vi "Autonomous Independent.vi"() -> ()   [LabVIEW 2013]
doc: "This VI is called when autonomous begins, and will automatically be terminated when autonomous ends. You can carry out timed or sensor driven robot movement independently without needing to return to the caller."
uses:
  Robot Global Data.vi
  <vilib>/Rock Robotics/WPI/RobotDrive/WPI_RobotDriveArcadeDrive_Standard(NoSaturation).vi
  <vilib>/Rock Robotics/WPI/RobotDrive/WPI_RobotDriveGetSetRefNum.vi
  <vilib>/Rock Robotics/WPI/Joystick/WPI_JoystickGetSetRefNum.vi
panel:
  out "Current Movement, for debugging":T1 {"Y Joystick Value" scale=1.0..-1.0; "X Joystick Value" scale=-1.0..1.0}
  in  "Array of robot movements":T2(array[cluster]) {"Y Joystick Value" scale=1.0..-1.0; "X Joystick Value" scale=-1.0..1.0}
  # "Be sure to right-click and choose Data Operations>>Make Current Value default if you want to save the array values with the VI"
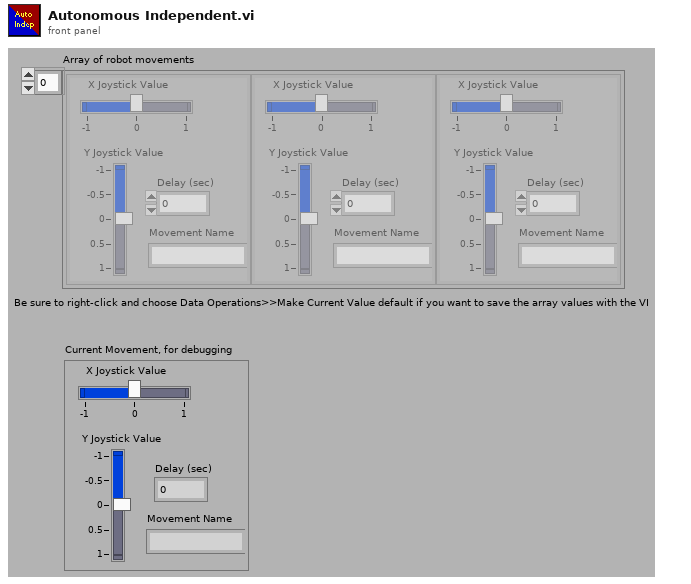
[diagram p1: front panel]
types:
  T1 = cluster{"X Joystick Value":dbl, "Y Joystick Value":dbl, "Delay (sec)":dbl, "Movement Name":string}
  T2 = cluster{"X Joystick Value":dbl, "Y Joystick Value":dbl, "Delay (sec)":dbl, "Movement Name":string}[]
  T3 = typedef "WPI_JoystickDevRef.ctl" = cluster{"Device":T4}
  T4 = typedef "WPI_JoystickDeviceEnum.ctl" = enum16{"USB 1", "USB 2", "USB 3", "USB 4", "Kinect 1", "Kinect 2"}
  T5 = cluster{"axis 1 (x)":dbl, "axis 2 (y)":dbl, "axis 3 (throttle)":dbl, "axis 4":dbl, "axis 5":dbl, "axis 6":dbl}
  T6 = typedef "WPI_RobotDriveDevRef.ctl" = cluster{"DevStatus":errorcluster, "Motors[]":T7[], "Square Inputs":bool, "Max Output":dbl, "Isochronous":bool}
  T7 = typedef "WPI_MotorControlDeviceRef.ctl" = cluster{"DeviceStatus":errorcluster, "Type":enum16{"PWM", "CAN"}, "PWM":cluster{"Digital Module":T8, "PWM Channel":T9, "DeadBand":T10}, "CAN":cluster{"Device Number":u8, "Control Mode":T11, "Semaphore":T12, "Max Vout":dbl}, "Invert":bool, "TransformRef":T13, "InvTransformRef":T13}
  T8 = typedef "FPGA_TypedefDigitalModule.ctl" = enum16{"Digital Module 1", "Digital Module 2"}
  T9 = typedef "FPGA_DIOPWMChannel.ctl" = enum8{"PWM 1", "PWM 2", "PWM 3", "PWM 4", "PWM 5", "PWM 6", "PWM 7", "PWM 8", "PWM 9", "PWM 10", "Invalid"}
  T10 = typedef "WPI_PWMDeadband.ctl" = cluster{"Name":string, "maxPositivePwm":i32, "minPositivePwm":i32, "centerPwm":i32, "maxNegativePwm":i32, "minNegativePwm":i32, "angularRange":u16}
  T11 = typedef "WPI_CANJaguar_ControlMode.ctl" = enum8{"Percent VBus", "Current", "Speed", "Position", "Voltage"}
  T12 = typedef "Semaphore RefNum" = refnum<k1>
  T13 = typedef "WPI_PWMTransform_ConPane.ctl" = refnum<vi>
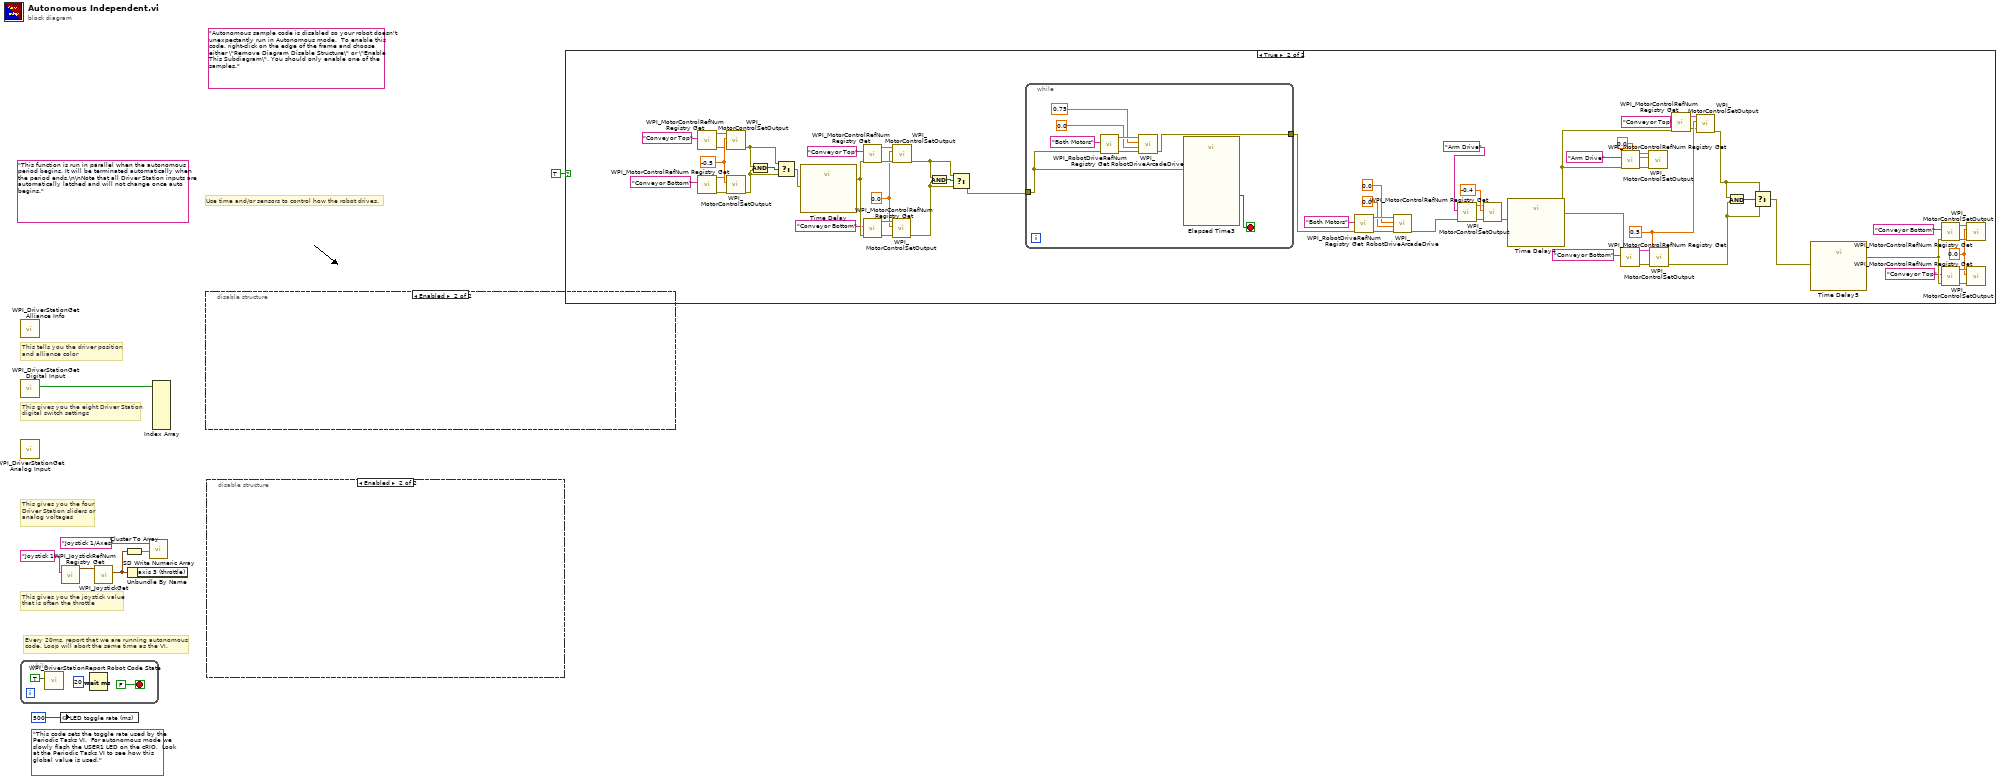
[diagram p0: block diagram]
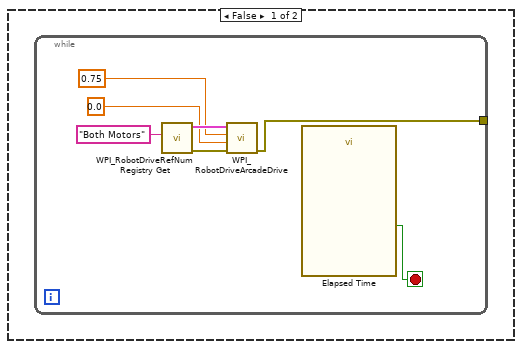
[diagram p2: hidden frame]
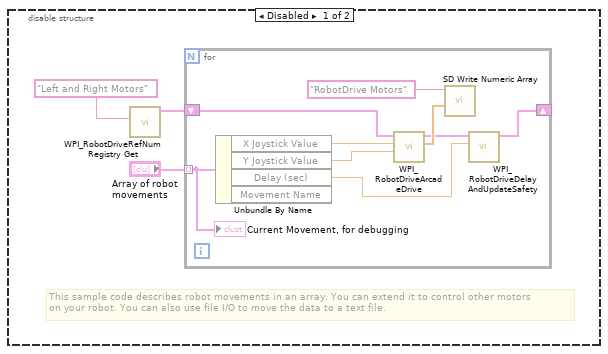
[diagram p3: hidden frame]
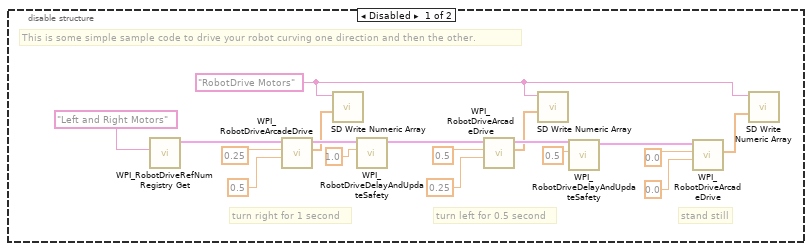
[diagram p4: hidden frame]
diagram:
  (unwired) "This code sets the toggle rate used by the Periodic Tasks VI.  For autonomous mode we slowly flash the USER1 LED on the cRIO.  Look at the Periodic Tasks VI to see how this global value is used."
  (unwired) "Autonomous sample code is disabled so your robot doesn't unexpectantly run in Autonomous mode.  To enable this code, right-click on the edge of the frame and choose either \"Remove Diagram Disable Structure\" or \"Enable This Subdiagram\". You should only enable one of the samples."
  (unwired) "This function is run in parallel when the autonomous period begins. It will be terminated automatically when the period ends.\n\nNote that all Driver Station inputs are automatically latched and will not change once auto begins."
  # "Every 20ms, report that we are running autonomous\ncode. Loop will abort the same time as the VI."
  # "This gives you the joystick value\nthat is often the throttle"
  # "Use time and/or sensors to control how the robot drives."
  # "This tells you the driver position\nand alliance color"
  # "This gives you the eight Driver Station\ndigital switch settings"
  # "This gives you the four\nDriver Station sliders or\nanalog voltages"
  n1 = while {
    stop <- FALSE stop-if-true
    n2 = call <vilib>:"WPI_DriverStationReport Robot Code State.vi"("Autonomous"=TRUE) -> ()  [unwired: 10 in, 1 out]
    n3 = Wait (ms)(milliseconds to wait=u32 20) -> ()  [unwired: 1 out]
  }
  n4 = call <vilib>:"WPI_DriverStationGet Alliance Info.vi"() -> ()  [unwired: 12 out]
  n5 = call <vilib>:"WPI_DriverStationGet Digital Input.vi"() -> ("Driver Station Digital Input (1-8)"=w8:bool[])  [unwired: 11 out]
  n6 = call <vilib>:"WPI_DriverStationGet Analog Input.vi"() -> ()  [unwired: 12 out]
  n7 = global write "Robot Global Data.vi" "LED toggle rate (ms)"(u32 500 ("LED ms toggle rate")) -> ()
  n8 = call <vilib>:"WPI_JoystickRefNum Registry Get.vi"("refnum name"="Joystick 1") -> ("JoystickDevRef"=w6:T3)  [unwired: 1 in, 9 out]
  n9 = call <vilib>:"WPI_JoystickGet.vi"("JoystickDevRef"=w6) -> ("Axes"=w3:T5)  [unwired: 1 in, 5 out]
  n10 = Cluster To Array(cluster=w3) -> (array=w4:dbl[])
  n11 = Unbundle By Name(w3) -> ()  [unwired: 1 out]
  n12 = call <vilib>:"SD Write Numeric Array.vi"("Numeric Array"=w4, "Name"="Joystick 1/Axes") -> ()  [unwired: 8 in, 2 out]
  n13 = Index Array(array=w8) -> ()  [unwired: 8 in, 8 out]
  n14 = disable-structure shown="Enabled" {
    frame Disabled {
      w12 = "RobotDrive Motors" ("Name")
      # "This is some simple sample code to drive your robot curving one direction and then the other."
      # "stand still"
      # "turn left for 0.5 second"
      # "turn right for 1 second"
      n15 = call <vilib>:"WPI_RobotDriveRefNum Registry Get.vi"("refnum name"="Left and Right Motors") -> ("RobotDriveDevRef"=w16:T6)  [unwired: 1 in, 9 out]
      n16 = call-poly <vilib>:"WPI_RobotDriveArcadeDrive.vi"("Y axis value"=0.5 ("X axis value"), "X axis value"=0.25, "RobotDriveDevRef"=w16) -> ("Motor Values"=w15:dbl[], "RobotDriveDevRef"=w23:T6)  [unwired: 1 in, 6 out]
      n17 = call <vilib>:"SD Write Numeric Array.vi"("Numeric Array"=w15, "Name"=w12) -> ()  [unwired: 8 in, 2 out]
      n18 = call <vilib>:"WPI_RobotDriveDelayAndUpdateSafety.vi"("Delay (s)"=1.0, "RobotDriveDevRef"=w23) -> ("RobotDriveDevRef 2"=w22:T6)  [unwired: 8 in, 1 out]
      n19 = call-poly <vilib>:"WPI_RobotDriveArcadeDrive.vi"("Y axis value"=0.25 ("X axis value"), "X axis value"=0.5, "RobotDriveDevRef"=w22) -> ("Motor Values"=w14:dbl[], "RobotDriveDevRef"=w21:T6)  [unwired: 1 in, 6 out]
      n20 = call <vilib>:"SD Write Numeric Array.vi"("Numeric Array"=w14, "Name"=w12) -> ()  [unwired: 8 in, 2 out]
      n21 = call <vilib>:"WPI_RobotDriveDelayAndUpdateSafety.vi"("Delay (s)"=0.5, "RobotDriveDevRef"=w21) -> ("RobotDriveDevRef 2"=w20:T6)  [unwired: 8 in, 1 out]
      n22 = call-poly <vilib>:"WPI_RobotDriveArcadeDrive.vi"("Y axis value"=0.0 ("X axis value"), "X axis value"=0.0, "RobotDriveDevRef"=w20) -> ("Motor Values"=w13:dbl[])  [unwired: 1 in, 7 out]
      n23 = call <vilib>:"SD Write Numeric Array.vi"("Numeric Array"=w13, "Name"=w12) -> ()  [unwired: 8 in, 2 out]
    }
    frame Enabled {
    }
  }
  n24 = disable-structure shown="Enabled" {
    frame Disabled {
      # "This sample code describes robot movements in an array. You can extend it to control other motors\non your robot. You can also use file I/O to move the data to a text file."
      n25 = call <vilib>:"WPI_RobotDriveRefNum Registry Get.vi"("refnum name"="Left and Right Motors") -> ("RobotDriveDevRef"=w31:T6)  [unwired: 1 in, 9 out]
      n26 = for {
        shift-right: [w37] -> _
        shift-left: w31 -> [w38]
        tunnel: "Array of robot movements" -> [w33] mode=indexing
        n27 = Unbundle By Name(w33) -> ("X Joystick Value"=w36:dbl, "Y Joystick Value"=w35:dbl, "Delay (sec)"=w34:dbl)  [unwired: 1 out]
        n28 = call-poly <vilib>:"WPI_RobotDriveArcadeDrive.vi"("Y axis value"=w35, "X axis value"=w36, "RobotDriveDevRef"=w38) -> ("Motor Values"=w40:dbl[], "RobotDriveDevRef"=w39:T6)  [unwired: 1 in, 6 out]
        n29 = call <vilib>:"SD Write Numeric Array.vi"("Numeric Array"=w40, "Name"="RobotDrive Motors") -> ()  [unwired: 8 in, 2 out]
        n30 = call <vilib>:"WPI_RobotDriveDelayAndUpdateSafety.vi"("Delay (s)"=w34, "RobotDriveDevRef"=w39) -> ("RobotDriveDevRef 2"=w37:T6)  [unwired: 8 in, 1 out]
        "Current Movement, for debugging" <- w33
      }
    }
    frame Enabled {
    }
  }
  n31 = case shown="True" TRUE {
    frame False {
      n32 = while {
        tunnel: [w42] -> _
        stop <- w43 stop-if-true
        n33 = call <vilib>:"WPI_RobotDriveRefNum Registry Get.vi"("refnum name"="Both Motors") -> ("error out"=w47:errorcluster, "RobotDriveDevRef"=w48:T6)  [unwired: 9 in]
        n34 = call-poly <vilib>:"WPI_RobotDriveArcadeDrive.vi"("error in (no error)"=w47, "Y axis value"=0.0, "X axis value"=0.75, "RobotDriveDevRef"=w48) -> ("error out"=w42:errorcluster)  [unwired: 5 in, 2 out]
        n35 = call "Elapsed Time"() -> ("Time has Elapsed"=w43:bool)  [unwired: 12 in, 7 out]
      }
    }
    frame True {
      w95 = 0.0 ("Output")
      w84 = 0.5 ("Output")
      w70 = 0.0 ("Output")
      w62 = -0.5 ("Output")
      n36 = call <vilib>:"WPI_MotorControlRefNum Registry Get.vi"("refnum name"="Conveyor Top") -> ("error out"=w58:errorcluster, "MotorControlDevRef"=w57:T7)  [unwired: 9 in]
      n37 = call <vilib>:"WPI_MotorControlRefNum Registry Get.vi"("refnum name"="Conveyor Bottom") -> ("error out"=w59:errorcluster, "MotorControlDevRef"=w60:T7)  [unwired: 9 in]
      n38 = call <vilib>:"WPI_MotorControlSetOutput.vi"("error in (no error)"=w58, "Output"=w62, "MotorControlDevRef"=w57) -> ("error out"=w64:errorcluster)  [unwired: 6 in, 2 out]
      n39 = call <vilib>:"WPI_MotorControlSetOutput.vi"("error in (no error)"=w59, "Output"=w62, "MotorControlDevRef"=w60) -> ("error out"=w65:errorcluster)  [unwired: 6 in, 2 out]
      n40 = And(x=w64, y=w65) -> (x .and. y?=w63:bool)
      n41 = Select(t=w64, s=w63, f=w65) -> (s? t:f=w66:errorcluster)
      n42 = call "Time Delay"("error in (no error)"=w66) -> ("error out"=w77:errorcluster)  [unwired: 10 in]
      n43 = call <vilib>:"WPI_MotorControlRefNum Registry Get.vi"("error in (no error)"=w77, "refnum name"="Conveyor Top") -> ("error out"=w74:errorcluster, "MotorControlDevRef"=w75:T7)  [unwired: 8 in]
      n44 = call <vilib>:"WPI_MotorControlRefNum Registry Get.vi"("error in (no error)"=w77, "refnum name"="Conveyor Bottom") -> ("error out"=w73:errorcluster, "MotorControlDevRef"=w72:T7)  [unwired: 8 in]
      n45 = call <vilib>:"WPI_MotorControlSetOutput.vi"("error in (no error)"=w73, "Output"=w70, "MotorControlDevRef"=w72) -> ("error out"=w67:errorcluster)  [unwired: 6 in, 2 out]
      n46 = call <vilib>:"WPI_MotorControlSetOutput.vi"("error in (no error)"=w74, "Output"=w70, "MotorControlDevRef"=w75) -> ("error out"=w68:errorcluster)  [unwired: 6 in, 2 out]
      n47 = And(x=w68, y=w67) -> (x .and. y?=w69:bool)
      n48 = Select(t=w68, s=w69, f=w67) -> (s? t:f=w106:errorcluster)
      n49 = while {
        tunnel: w106 -> [w109]
        tunnel: [w108] -> w54
        stop <- w110 stop-if-true
        n50 = call <vilib>:"WPI_RobotDriveRefNum Registry Get.vi"("error in (no error)"=w109, "refnum name"="Both Motors") -> ("error out"=w114:errorcluster, "RobotDriveDevRef"=w115:T6)  [unwired: 8 in]
        n51 = call-poly <vilib>:"WPI_RobotDriveArcadeDrive.vi"("error in (no error)"=w114, "Y axis value"=0.0, "X axis value"=0.75, "RobotDriveDevRef"=w115) -> ("error out"=w108:errorcluster)  [unwired: 5 in, 2 out]
        n52 = call "Elapsed Time3"("error in (no error)"=w109) -> ("Time has Elapsed"=w110:bool)  [unwired: 11 in, 7 out]
      }
      n53 = call <vilib>:"WPI_RobotDriveRefNum Registry Get.vi"("error in (no error)"=w54, "refnum name"="Both Motors") -> ("error out"=w52:errorcluster, "RobotDriveDevRef"=w53:T6)  [unwired: 8 in]
      n54 = call-poly <vilib>:"WPI_RobotDriveArcadeDrive.vi"("error in (no error)"=w52, "Y axis value"=0.0, "X axis value"=0.0, "RobotDriveDevRef"=w53) -> ("error out"=w107:errorcluster)  [unwired: 5 in, 2 out]
      n55 = call <vilib>:"WPI_MotorControlRefNum Registry Get.vi"("error in (no error)"=w107, "refnum name"="Arm Drive") -> ("error out"=w88:errorcluster, "MotorControlDevRef"=w89:T7)  [unwired: 8 in]
      n56 = call <vilib>:"WPI_MotorControlSetOutput.vi"("error in (no error)"=w88, "Output"=-0.4 ("t"), "MotorControlDevRef"=w89) -> ("error out"=w90:errorcluster)  [unwired: 6 in, 2 out]
      n57 = call "Time Delay4"("error in (no error)"=w90) -> ("error out"=w105:errorcluster)  [unwired: 10 in]
      n58 = call <vilib>:"WPI_MotorControlRefNum Registry Get.vi"("error in (no error)"=w105, "refnum name"="Conveyor Bottom") -> ("error out"=w81:errorcluster, "MotorControlDevRef"=w82:T7)  [unwired: 8 in]
      n59 = call <vilib>:"WPI_MotorControlRefNum Registry Get.vi"("error in (no error)"=w105, "refnum name"="Arm Drive") -> ("error out"=w93:errorcluster, "MotorControlDevRef"=w92:T7)  [unwired: 8 in]
      n60 = call <vilib>:"WPI_MotorControlSetOutput.vi"("error in (no error)"=w93, "Output"=0.0, "MotorControlDevRef"=w92) -> ()  [unwired: 6 in, 3 out]
      n61 = call <vilib>:"WPI_MotorControlSetOutput.vi"("error in (no error)"=w81, "Output"=w84, "MotorControlDevRef"=w82) -> ("error out"=w87:errorcluster)  [unwired: 6 in, 2 out]
      n62 = call <vilib>:"WPI_MotorControlRefNum Registry Get.vi"("error in (no error)"=w105, "refnum name"="Conveyor Top") -> ("error out"=w80:errorcluster, "MotorControlDevRef"=w79:T7)  [unwired: 8 in]
      n63 = call <vilib>:"WPI_MotorControlSetOutput.vi"("error in (no error)"=w80, "Output"=w84, "MotorControlDevRef"=w79) -> ("error out"=w86:errorcluster)  [unwired: 6 in, 2 out]
      n64 = And(x=w86, y=w87) -> (x .and. y?=w85:bool)
      n65 = Select(t=w86, s=w85, f=w87) -> (s? t:f=w94:errorcluster)
      n66 = call "Time Delay5"("error in (no error)"=w94) -> ("error out"=w102:errorcluster)  [unwired: 10 in]
      n67 = call <vilib>:"WPI_MotorControlRefNum Registry Get.vi"("error in (no error)"=w102, "refnum name"="Conveyor Bottom") -> ("error out"=w98:errorcluster, "MotorControlDevRef"=w97:T7)  [unwired: 8 in]
      n68 = call <vilib>:"WPI_MotorControlRefNum Registry Get.vi"("error in (no error)"=w102, "refnum name"="Conveyor Top") -> ("error out"=w99:errorcluster, "MotorControlDevRef"=w100:T7)  [unwired: 8 in]
      n69 = call <vilib>:"WPI_MotorControlSetOutput.vi"("error in (no error)"=w98, "Output"=w95, "MotorControlDevRef"=w97) -> ()  [unwired: 6 in, 3 out]
      n70 = call <vilib>:"WPI_MotorControlSetOutput.vi"("error in (no error)"=w99, "Output"=w95, "MotorControlDevRef"=w100) -> ()  [unwired: 6 in, 3 out]
    }
  }
